vi "test single REQ.vi"() -> ()   [LabVIEW 2018, in "LV-Julia_ZMQ-Roundtrip_lib.lvlib"]
uses:
  LV-Julia_ZMQ-Roundtrip_lib.lvlib
  Commands v2.ctl
panel:
  out "server response":string
  in  "data to send":string="hello"
  out "error out":errorcluster
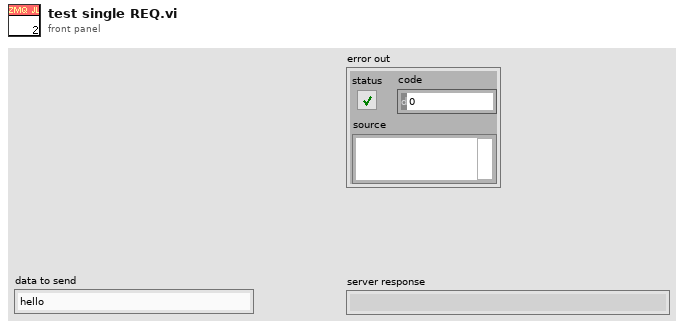
[diagram p1: front panel]
types:
  T1 = typedef "LV-Julia_ZMQ-Roundtrip_lib.lvlib/Commands v2.ctl" = enum16{"Start Jl-server & Init LV-client", "Send request & Get response ", "Stop Jl-server & Cleanup LV-client", "Cleanup LV-client", "Start Jl-server", "Stop Jl-server", "Init LV-Client", "Cleanup LV-Client", "(not allowed)", "Set LV Client state", "Set Jl Server state"}
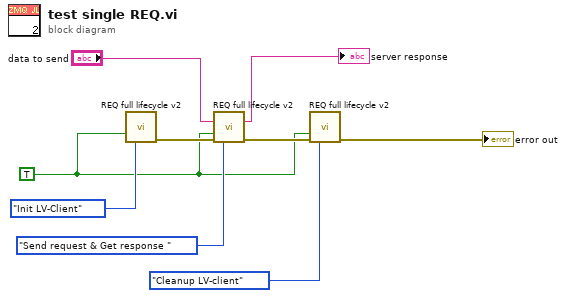
[diagram p0: block diagram]
diagram:
  w3 = TRUE ("Force command")
  n1 = call "REQ full lifecycle v2.vi"("Force command"=w3, "command"=Commands_v2."Init LV-Client") -> ("error out"=w8:errorcluster)  [unwired: 10 in, 3 out]
  n2 = call "REQ full lifecycle v2.vi"("data to send"="data to send", "Force command"=w3, "error in"=w8, "command"=Commands_v2."Send request & Get response ") -> ("server response"=→"server response":string, "error out"=w6:errorcluster)  [unwired: 8 in, 2 out]
  n3 = call "REQ full lifecycle v2.vi"("Force command"=w3, "error in"=w6, "command"=Commands_v2."Cleanup LV-client") -> ("error out"=→"error out":errorcluster)  [unwired: 9 in, 3 out]
